vi "Find Entity by ID.vi"(6 "Entity ID":T1, 7 "Entity Type":refnum<class "Entity.lvclass">, 8 "error in (no error)":errorcluster, 9 "Database in":refnum<class "Database Platform.lvclass">, 10 "Types":refnum<class "Type.lvclass">[](array[class]), 11 "Unit Of Work in":refnum<class "Unit Of Work Session.lvclass">) -> (0 "error out":errorcluster, 1 "Database out":refnum<class "Database Platform.lvclass">, 2 "Entity":refnum<class "Entity.lvclass">)   [LabVIEW 2020, in "Conditu2.lvlib" / "Unit Of Work Session.lvclass"]
uses:
  Unit Of Work Session.lvclass
  Database Platform/Database Platform.lvclass
  Entity/Entity.lvclass
  Entity ID.ctl
  Columns/Type/Type.lvclass
  Unit Of Work Session.lvclass/Unit Of Work Session.ctl
  <vilib>/Utility/miscctls.llb/LVMapReplaceAction.ctl
  Conditu2.lvlib
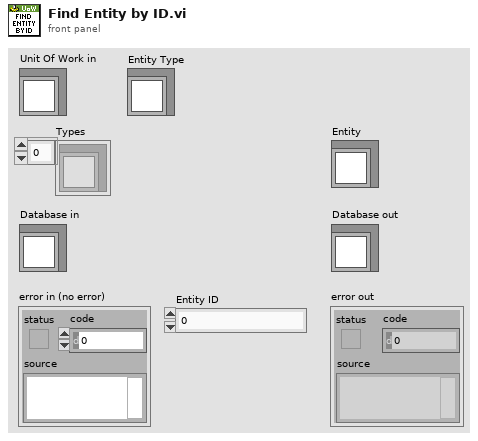
[diagram p1: front panel]
types:
  T1 = typedef "Conditu2.lvlib/Entity ID.ctl" = i64
  T2 = typedef "LVMapReplaceAction.ctl" = enum32{"Modify Entry only if found", "Add or Modify Entry", "Delete Entry"}
  T3 = typedef "Conditu2.lvlib/Unit Of Work Session.lvclass/Ref Data.ctl" = cluster{"Entity Class Map":T4}
  T4 = typedef "Conditu2.lvlib/Unit Of Work Session.lvclass/Entity Class Map.ctl" = map{string, map{T1, refnum<class "Entity.lvclass">}}
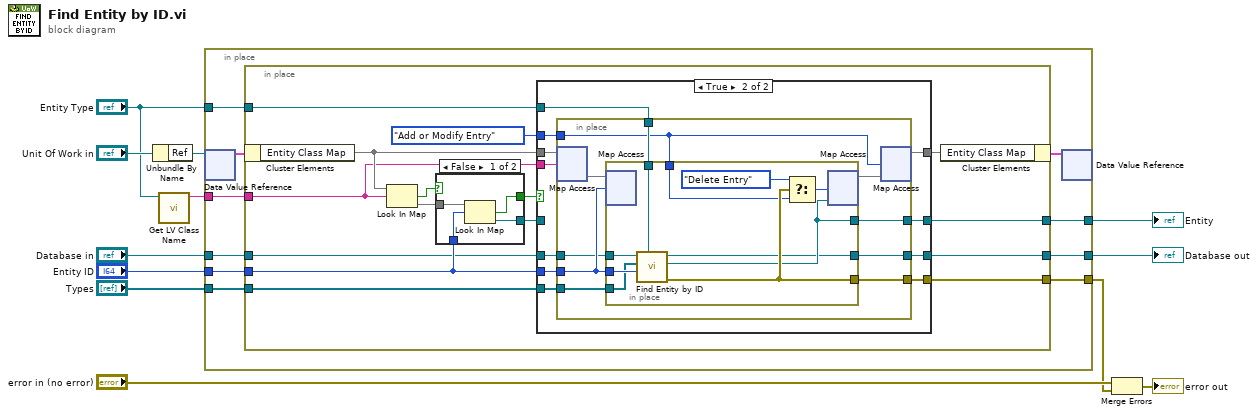
[diagram p0: block diagram]
diagram:
  n1 = Unbundle By Name("Unit Of Work in") -> ("Ref"=w11:refnum<data-value>)
  n2 = call <vilib>:"Get LV Class Name.vi"("object"="Entity Type") -> ("class name"=w10:string)  [unwired: 9 in, 1 out]
  n3 = in-place {
    in-place-border: w10 -> [w21]
    in-place-border: "Entity ID" -> [w19]
    in-place-border: [w18] -> w8
    in-place-border: "Database in" -> [w17]
    in-place-border: "Entity Type" -> [w16]
    in-place-border: "Types" -> [w15]
    in-place-border: [w14] -> w4
    in-place-border: [w13] -> w1
    n4 = in-place-dvr #1(w11) -> (w22:T3)  [unwired: 1 out]
    n5 = in-place {
      in-place-border: w21 -> [w30]
      in-place-border: w19 -> [w29]
      in-place-border: [w33] -> w18
      in-place-border: w17 -> [w28]
      in-place-border: w16 -> [w27]
      in-place-border: w15 -> [w26]
      in-place-border: [w24] -> w14
      in-place-border: [w23] -> w13
      n6 = in-place-cluster #2(w22) -> ("Entity Class Map"=w32:T4)
      n7 = Look In Map(map=w32, key=w30) -> (key not found?=w37:bool, value=w36:map{T1, refnum<class "Entity.lvclass">})  [unwired: 1 in]
      n8 = case shown="False" w37 {
        selector: w37 -> [_ w76]
        tunnel: w36 -> [w75 _]
        tunnel: w29 -> [w74 _]
        tunnel: [w73 _] -> w34
        tunnel: [w72 w76] -> w35
        frame False {
          n9 = Look In Map(map=w75, key=w74) -> (key not found?=w72:bool, value=w73:refnum<class "Entity.lvclass">)  [unwired: 1 in]
        }
        frame True {
        }
      }
      n10 = case shown="True" w35 {
        tunnel: w34 -> [w40 _]
        tunnel: [w40 w44] -> w33
        tunnel: w32 -> [w39 w51]
        tunnel: [w39 w43] -> w31
        tunnel: w30 -> [_ w50]
        tunnel: w29 -> [_ w49]
        tunnel: w28 -> [w38 w48]
        tunnel: w27 -> [_ w47]
        tunnel: w26 -> [_ w46]
        tunnel: LVMapReplaceAction."Add or Modify Entry" ("action") -> [_ w45]
        tunnel: [w38 w42] -> w24
        tunnel: [_ w41] -> w23
        frame False {
        }
        frame True {
          n11 = in-place {
            in-place-border: w49 -> [w60]
            in-place-border: w48 -> [w59]
            in-place-border: w47 -> [w58]
            in-place-border: w46 -> [w57]
            in-place-border: w45 -> [w52]
            in-place-border: [w56] -> w44
            in-place-border: [w54] -> w42
            in-place-border: [w53] -> w41
            n12 = in-place-map #3(w51, w50) -> (w61:map{T1, refnum<class "Entity.lvclass">})  [unwired: 1 in, 1 out]
            n13 = in-place {
              in-place-border: w60 -> [w70]
              in-place-border: w59 -> [w69]
              in-place-border: w58 -> [w68]
              in-place-border: w57 -> [w67]
              in-place-border: [w66] -> w56
              in-place-border: [w65] -> w54
              in-place-border: [w71] -> w53
              in-place-border: w52 -> [w62]
              n14 = in-place-map #4(w61, w60) -> ()  [unwired: 1 in, 2 out]
              n15 = call "Find Entity by ID.vi"("Entity Type"=w68, "Entity ID"=w70, "Types"=w67, "Database in"=w69) -> ("error out"=w71:errorcluster, "Entity"=w66:refnum<class "Entity.lvclass">, "Database out"=w65:refnum<class "Database Platform.lvclass">)  [unwired: 5 in]
              n16 = Select(t=LVMapReplaceAction."Delete Entry" ("action"), s=w71, f=w62) -> (s? t:f=w63:T2)
              n17 = in-place-map #4(w66, w63) -> (w55:map{T1, refnum<class "Entity.lvclass">})  [unwired: 2 out]
            }
            n18 = in-place-map #3(w55, w52) -> (w43:T4)  [unwired: 2 out]
          }
        }
      }
      n19 = in-place-cluster #2("Entity Class Map"=w31) -> (w20:T3)
    }
    n20 = in-place-dvr #1(w20) -> ()  [unwired: 2 out]
  }
  "Database out" <- w4
  "Entity" <- w8
  n21 = Merge Errors("error in (no error)", w1) -> (→"error out":errorcluster)
